vi "UART.vi"() -> ()   [LabVIEW 2018]
uses:
  <vilib>/myRIO/Instrument Drivers/Onboard IO/UART/typedef/VISA Configuration.ctl
  <vilib>/Instr/_visa.llb/VISA Configure Serial Port (Instr).vi
  <vilib>/myRIO/Express VI/Onboard IO/UART/UART Express VI.xnode
  <vilib>/myRIO/Instrument Drivers/Onboard IO/UART/UART.lvlib
panel:
  out "Characters Read":string
  out "s? t:f":string[](array[string])
  in  "stop":bool
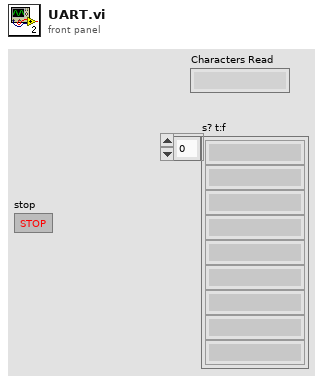
[diagram p1: front panel]
types:
  T1 = typedef "UART.lvlib/VISA Configuration.ctl" = cluster{"baud rate (9600)":u32, "data bits (8)":u16, "parity (0:none)":enum16{"None", "Odd", "Even", "Mark", "Space"}, "stop bits (10: 1 bit)":u16, "flow control (0:none)":u16, "termination char\n(0xA = '\\n' = LF) ":u8, "Enable Termination\nChar (T)":bool, "timeout (10sec)":u32}
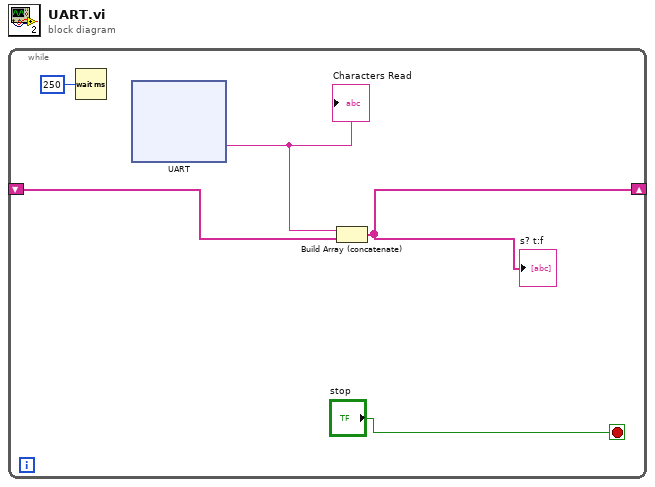
[diagram p0: block diagram]
diagram:
  n1 = while {
    shift-right: [w1] -> _
    shift-left: _ -> [w2]
    stop <- "stop" stop-if-true
    n2 = Wait (ms)(milliseconds to wait=u32 250) -> ()  [unwired: 1 out]
    n3 = xnode "UART"() -> ("Characters Read"=w4:string)  [unwired: 1 in, 1 out]
    "Characters Read" <- w4
    n4 = Build Array (concatenate)(w4, w2) -> (w1:string[])
    "s? t:f" <- w1
  }
